vi "Calculate Response Internal.vi"(10 "Inputs":dbl[](array[numeric]), 11 "Neural Network In":refnum<class "Neural Network.lvclass">) -> (0 "All Inputs":T1[](array[typedef]), 1 "Derrivatives":T1[](array[typedef]), 2 "Outputs":dbl[](array[numeric]), 3 "Neural Network Out":refnum<class "Neural Network.lvclass">)   [LabVIEW 2015, in "Neural Network.lvclass"]
uses:
  Neural Network.lvclass
  <vilib>/Analysis/NI_AALBase.lvlib
  <vilib>/Analysis/baseanly.llb/A x Vector.vi
  Types/1D Array.ctl
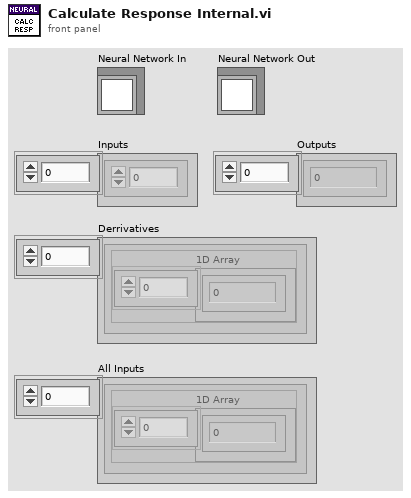
[diagram p1: front panel]
types:
  T1 = typedef "Neural Network.lvclass/1D Array.ctl" = cluster{"1D Array":dbl[]}
  T2 = typedef "Neural Network.lvclass/Scaling Info.ctl" = cluster{"X Scaling Vector":dbl[], "Y Scaling Vector":dbl[]}
  T3 = typedef "Neural Network.lvclass/2D Array.ctl" = cluster{"2D Array":sgl[][]}
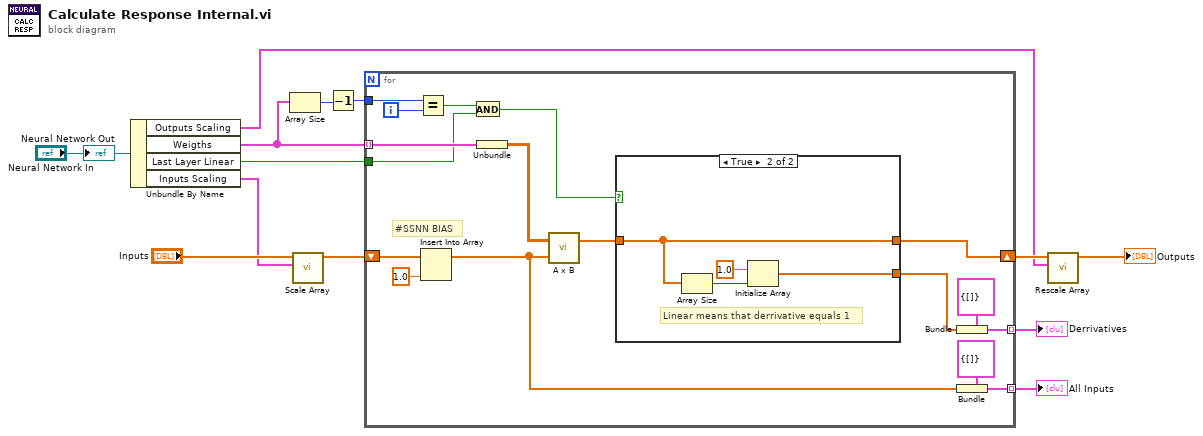
[diagram p0: block diagram]
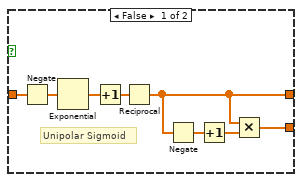
[diagram p2: hidden frame]
diagram:
  n1 = Unbundle By Name("Neural Network In") -> ("Outputs Scaling"=w1:T2, "Weigths"=w9:T3[], "Last Layer Linear"=w8:bool, "Inputs Scaling"=w5:T2)
  n2 = Array Size(array=w9) -> (size(s)=w11:i32)
  n3 = call "Scale Array.vi"("Scaling Info"=w5, "Array to Scale"="Inputs") -> ("Scaled Array"=w6:dbl[])  [unwired: 9 in]
  n4 = Decrement(x=w11) -> (x-1=w10:i32)
  n5 = for {
    shift-right: [w24] -> w4
    shift-left: w6 -> [w23]
    tunnel: [w28] -> w13 mode=indexing
    tunnel: w9 -> [w30] mode=indexing
    tunnel: [w27] -> w12 mode=indexing
    tunnel: w10 -> [w20]
    tunnel: w8 -> [w16]
    i -> [w18]
    # "#SSNN BIAS"
    n6 = Equal?(x=w20, y=w18) -> (x = y?=w19:bool)
    n7 = Insert Into Array(array=w23, new element=1.0 ("new element/subarray")) -> (w22:dbl[])  [unwired: 1 in]
    n8 = And(x=w19, y=w16) -> (x .and. y?=w17:bool)
    n9 = Unbundle(w30) -> ("2D Array"=w29:sgl[][])
    n10 = call-poly <vilib>:"A x B.vi"("Vector"=w22, "A"=w29) -> ("A x Vector"=w21:dbl[])  [unwired: 1 out]
    n11 = case shown="True" w17 {
      tunnel: [w33 w40] -> w25
      tunnel: [w32 w42] -> w24
      tunnel: w21 -> [w31 w42]
      frame False {
        # "Unipolar Sigmoid"
        n12 = Negate(x=w31) -> (-x=w38:dbl[])
        n13 = Exponential(1:w38) -> (0:w37:dbl[])
        n14 = Increment(x=w37) -> (x+1=w36:dbl[])
        n15 = Reciprocal(x=w36) -> (1/x=w32:dbl[])
        n16 = Negate(x=w32) -> (-x=w35:dbl[])
        n17 = Increment(x=w35) -> (x+1=w34:dbl[])
        n18 = Multiply(x=w32, y=w34) -> (x*y=w33:dbl[])
      }
      frame True {
        # "Linear means that derrivative equals 1"
        n19 = Array Size(array=w42) -> (size(s)=w41:i32)
        n20 = Initialize Array(1.0 ("new element/subarray"), w41) -> (w40:dbl[])
      }
    }
    n21 = Bundle(cluster=T1 {"1D Array"=[]} ("1D Array"), "1D Array"=w25) -> (w28:T1)
    n22 = Bundle(cluster=T1 {"1D Array"=[]} ("1D Array"), "1D Array"=w22) -> (w27:T1)
  }
  "Derrivatives" <- w13
  "All Inputs" <- w12
  n23 = call "Rescale Array.vi"("Scaling Info"=w1, "Array to Rescale"=w4) -> ("Rescaled Array"=→"Outputs":dbl[])  [unwired: 9 in]
  "Neural Network Out" <- "Neural Network In"
